vi "Reorder Driver Alias Array.vi"(8 "error in (no error)":errorcluster, 9 "New indices":u32[](array[numeric]), 10 "Driver Name":string, 11 "Instrument Handler in":refnum<class "Instrument Handler.lvclass">) -> (0 "error out":errorcluster, 1 "Success?":bool, 3 "Instrument Handler out":refnum<class "Instrument Handler.lvclass">)   [LabVIEW 2020, in "Instrument Handler.lvlib" / "Instrument Handler.lvclass"]
doc: "Reorder the Alias' associatied with 'Driver name'."
uses:
  Instrument Handler.lvclass
  Instrument Handler.lvclass/Instrument Handler.ctl
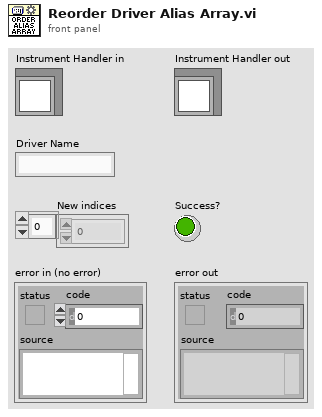
[diagram p1: front panel]
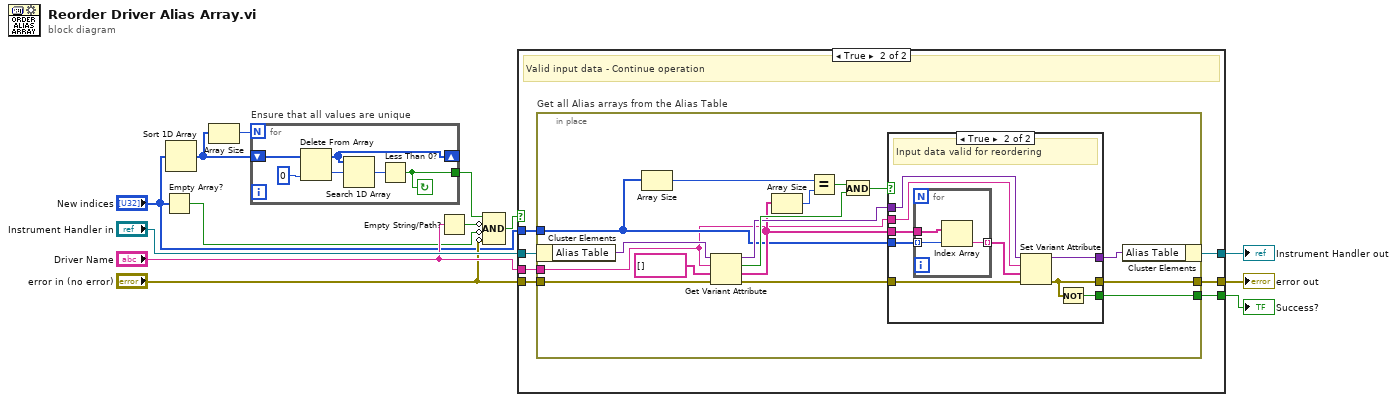
[diagram p0: block diagram]
diagram:
  n1 = Empty Array?(array="New indices") -> (empty?=w8:bool)
  n2 = Sort 1D Array(array="New indices") -> (sorted array=w4:u32[])
  n3 = Array Size(array=w4) -> (size(s)=w5:i32)
  n4 = for "Ensure that all values are unique" {
    N: w5 -> [_]
    shift-right: [w15] -> _
    shift-left: w4 -> [w19]
    tunnel: [w14] -> w2
    stop <- w14 continue-if-true
    n5 = Delete From Array(array=w19, index=0) -> (deleted portion=w17:u32, array with subset deleted=w15:u32[])  [unwired: 1 in]
    n6 = Search 1D Array(1D array=w15, element=w17) -> (index of element=w16:i32)  [unwired: 1 in]
    n7 = Less Than 0?(x=w16) -> (x < 0?=w14:bool)
  }
  n8 = Empty String/Path?(string/path="Driver Name") -> (empty?=w9:bool)
  n9 = Compound Arithmetic op=AND(w2, invert w9, invert w8, invert "error in (no error)") -> (w6:bool)
  n10 = case shown="True" w6 {
    tunnel: [w20 w26] -> w13
    tunnel: [w21 w22] -> w11
    tunnel: "Instrument Handler in" -> [w21 w23]
    tunnel: "Driver Name" -> [_ w28]
    tunnel: "error in (no error)" -> [w20 w27]
    tunnel: "New indices" -> [_ w25]
    tunnel: [_ w24] -> w1
    frame False {
      # "Invalid input data - Abort operation"
    }
    frame True {
      # "Valid input data - Continue operation"
      n11 = in-place "Get all Alias arrays from the Alias Table" {
        in-place-border: w27 -> [w43]
        in-place-border: w28 -> [w30]
        in-place-border: [w38] -> w26
        in-place-border: w25 -> [w31]
        in-place-border: [w29] -> w24
        n12 = in-place-cluster #1(w23) -> ("Alias Table"=w44:variant)
        n13 = Array Size(array=w31) -> (size(s)=w35:i32)
        n14 = Get Variant Attribute(Variant=w44, name=w30, default value (empty Variant)=string[] [] ("Driver Name"), error in=w43) -> (duplicate Variant=w39:variant, found=w41:bool, value=w36:string[], error out=w37:errorcluster)
        n15 = Array Size(array=w36) -> (size(s)=w34:i32)
        n16 = Equal?(x=w35, y=w34) -> (x = y?=w32:bool)
        n17 = And(x=w32, y=w41) -> (x .and. y?=w33:bool)
        n18 = case shown="True" w33 {
          tunnel: [w46 w49] -> w40
          tunnel: w39 -> [w46 w53]
          tunnel: [w45 w48] -> w38
          tunnel: w37 -> [w45 w50]
          tunnel: w36 -> [_ w55]
          tunnel: w31 -> [_ w54]
          tunnel: w30 -> [_ w52]
          tunnel: [_ w47] -> w29
          frame False {
            # "None or invalid data - Abort"
          }
          frame True {
            # "Input data valid for reordering"
            n19 = for {
              tunnel: w55 -> [w58]
              tunnel: w54 -> [w57] mode=indexing
              tunnel: [w56] -> w51 mode=indexing
              n20 = Index Array(array=w58, index=w57) -> (element=w56:string)
            }
            n21 = Set Variant Attribute(Variant=w53, name=w52, value=w51, error in=w50) -> (Variant out=w49:variant, error out=w48:errorcluster)  [unwired: 1 out]
            n22 = Not(x=w48) -> (.not. x?=w47:bool)
          }
        }
        n23 = in-place-cluster #1("Alias Table"=w40) -> (w22:refnum<class "Instrument Handler.lvclass">)
      }
    }
  }
  "error out" <- w13
  "Instrument Handler out" <- w11
  "Success?" <- w1
